vi "Equilibrium (SubVI).vi"(0 "Right":dbl, 1 "Left":dbl, 2 "Left Output":dbl, 3 "Right Output":dbl) -> (7 "Left Output New":dbl, 8 "Right Output New":dbl)   [LabVIEW 2017]
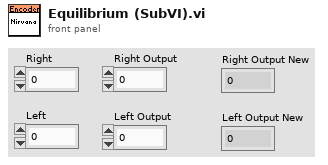
[diagram p1: front panel]
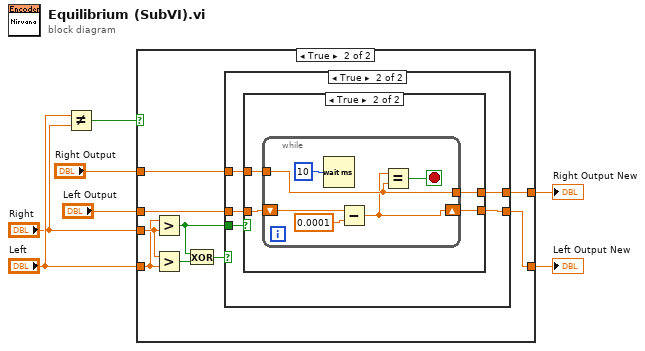
[diagram p0: block diagram]
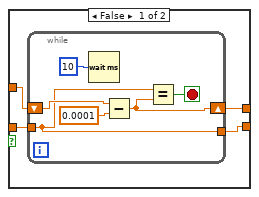
[diagram p4: hidden frame]
diagram:
  n1 = Not Equal?(x="Left", y="Right") -> (x != y?=w7:bool)
  n2 = case shown="True" w7 {
    tunnel: "Left" -> [w9 w17]
    tunnel: "Right" -> [_ w18]
    tunnel: "Left Output" -> [_ w13]
    tunnel: "Right Output" -> [w8 w12]
    tunnel: [w9 w11] -> w2
    tunnel: [w8 w10] -> w1
    frame False {
    }
    frame True {
      n3 = Greater?(x=w17, y=w18) -> (0:w14:bool)
      n4 = Greater?(x=w18, y=w17) -> (0:w16:bool)
      n5 = Exclusive Or(1:w16, 2:w14) -> (0:w15:bool)
      n6 = case shown="True" w15 {
        tunnel: w14 -> [_ w25]
        tunnel: w13 -> [w20 w24]
        tunnel: w12 -> [w19 w23]
        tunnel: [w20 w22] -> w11
        tunnel: [w19 w21] -> w10
        frame False {
        }
        frame True {
          n7 = case shown="True" w25 {
            tunnel: w24 -> [w28 w39]
            tunnel: w23 -> [w29 w38]
            tunnel: [w27 w37] -> w21
            tunnel: [w26 w36] -> w22
            frame False {
              n8 = while {
                tunnel: w28 -> [w32]
                tunnel: [w32] -> w26
                shift-right: [w33] -> w27
                shift-left: w29 -> [w35]
                stop <- w34 stop-if-true
                n9 = Wait (ms)(milliseconds to wait=u32 10) -> ()  [unwired: 1 out]
                n10 = Subtract(x=w35, y=0.0001) -> (x-y=w33:dbl)
                n11 = Equal?(x=w32, y=w33) -> (x = y?=w34:bool)
              }
            }
            frame True {
              n12 = while {
                tunnel: w38 -> [w42]
                tunnel: [w42] -> w37
                shift-right: [w41] -> w36
                shift-left: w39 -> [w45]
                stop <- w43 stop-if-true
                n13 = Wait (ms)(milliseconds to wait=u32 10) -> ()  [unwired: 1 out]
                n14 = Subtract(x=w45, y=0.0001) -> (x-y=w41:dbl)
                n15 = Equal?(x=w41, y=w42) -> (x = y?=w43:bool)
              }
            }
          }
        }
      }
    }
  }
  "Left Output New" <- w2
  "Right Output New" <- w1
